vi "ExposeMapperToObjectNamepathDataRecursiverIterator.vi"(8 "BaseName":string, 9 "Skip Parent Name (t)":bool=TRUE, 11 "Value Reference In":refnum<data-value>) -> (2 "Object map":T1[](array[typedef]), 3 "Value Reference Out":refnum<data-value>)   [LabVIEW 2017]
uses:
  ExposeObjectMapNamepathData.ctl
  ExposeMapperDataTypeEnum.ctl
  ExposeObjectMapContainerTypeEnum.ctl
  ExposeMapperObjectTypeEnum.ctl
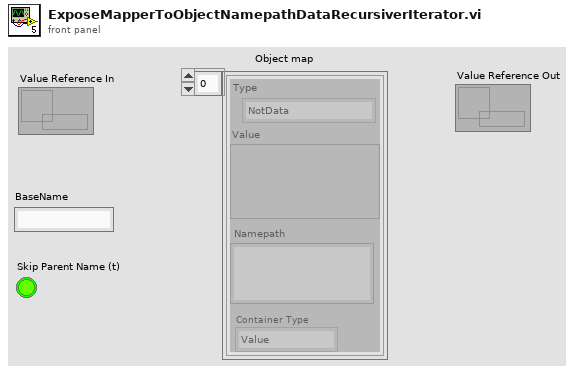
[diagram p1: front panel]
types:
  T1 = typedef "ExposeObjectMapNamepathData.ctl" = cluster{"Type":T2, "Value":variant, "Namepath":string, "Container Type":T3}
  T2 = typedef "ExposeMapperDataTypeEnum.ctl" = enum16{"NotData", "int8", "byte", "int16", "uint16", "int32", "uint32", "int64", "uint64", "Single", "Double", "String", "Boolean", "Container"}
  T3 = typedef "ExposeObjectMapContainerTypeEnum.ctl" = enum16{"Value", "Array", "Waveform", "NetContainer"}
  T4 = typedef "ExposeMapperObjectTypeEnum.ctl" = enum16{"NotAValidObject", "Value", "Variant", "Cluster", "Array", "Asng. Refnum"}
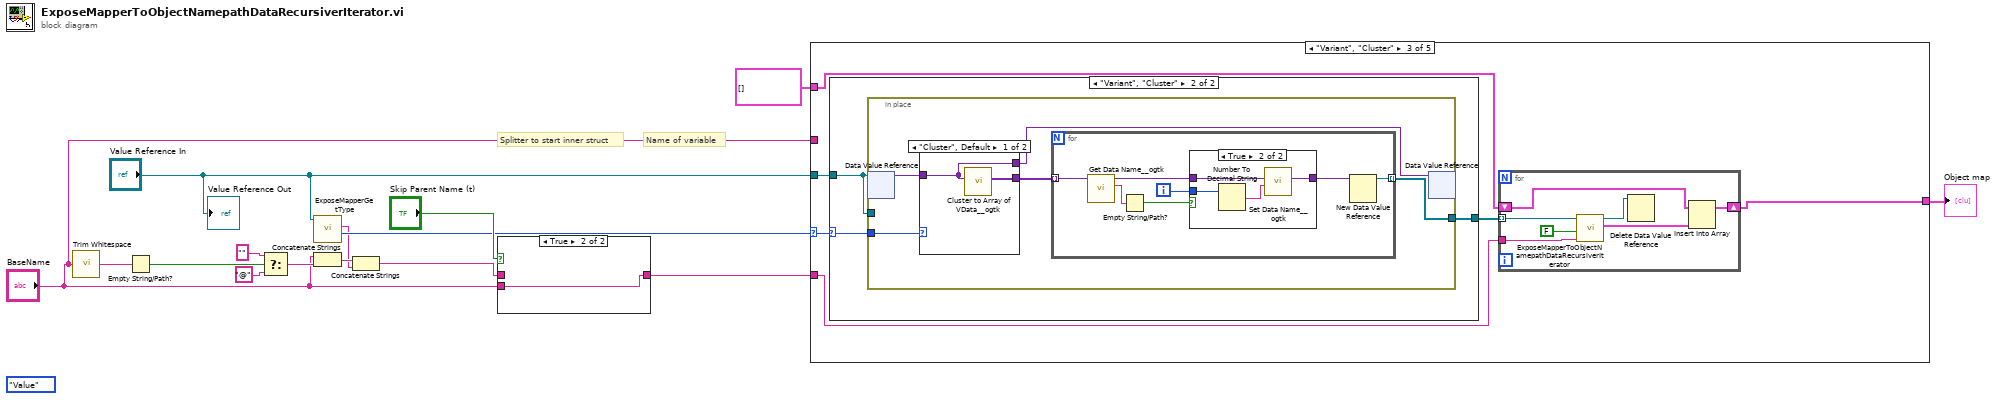
[diagram p0: block diagram]
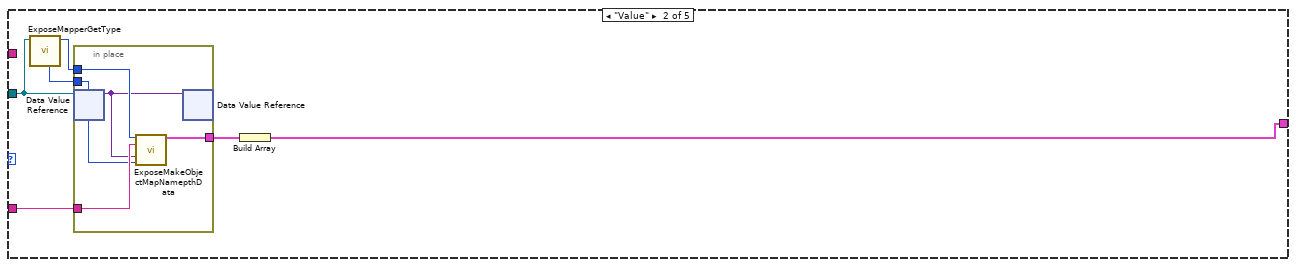
[diagram p4: hidden frame]
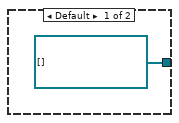
[diagram p5: hidden frame]
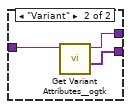
[diagram p6: hidden frame]
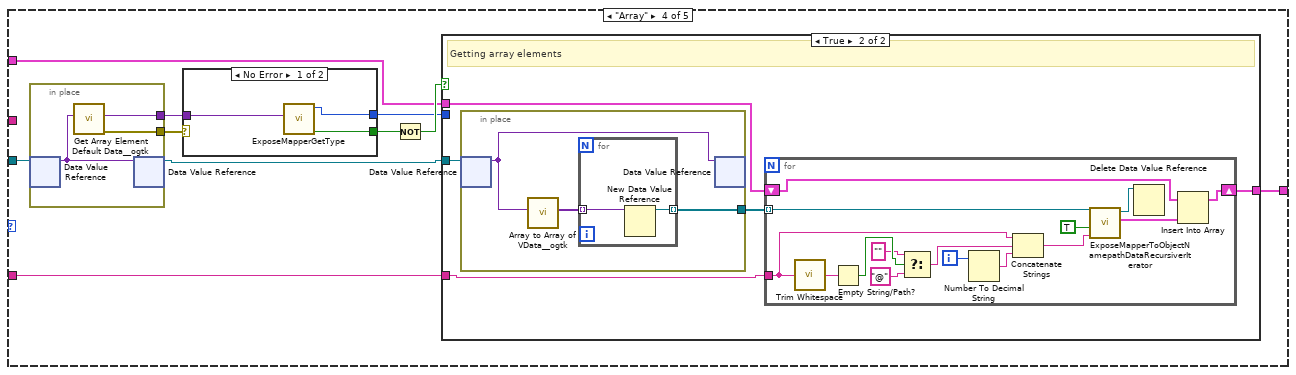
[diagram p8: hidden frame]
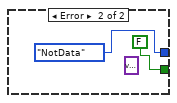
[diagram p9: hidden frame]
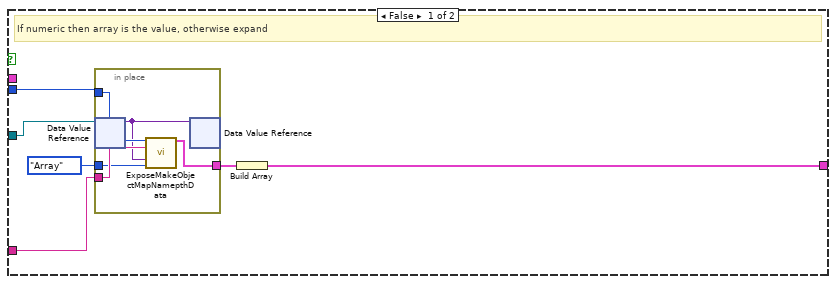
[diagram p10: hidden frame]
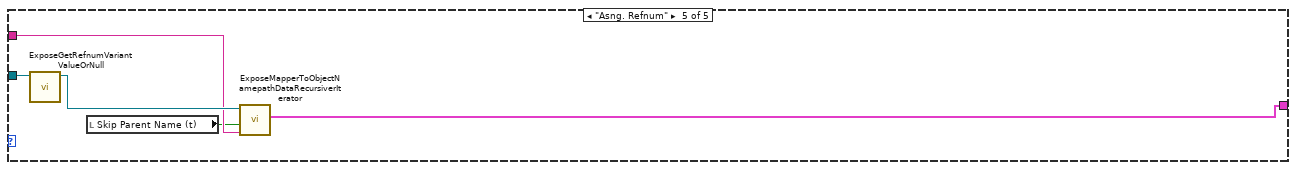
[diagram p11: hidden frame]
diagram:
  (unwired) ExposeMapperObjectTypeEnum."Value" ("OType")
  # "Splitter to start inner struct"
  # "Name of variable"
  n1 = call <vilib>:"Trim Whitespace.vi"("string"="BaseName") -> ("trimmed string"=w8:string)  [unwired: 1 in]
  n2 = Empty String/Path?(string/path=w8) -> (empty?=w7:bool)
  n3 = Select(t="" ("name"), s=w7, f="@" ("name")) -> (s? t:f=w15:string)
  n4 = call "ExposeMapperGetType.vi"("Data Val Ref in"="Value Reference In") -> ("OType"=w3:T4, "Name"=w2:string)  [unwired: 5 in, 4 out]
  n5 = Concatenate Strings("BaseName", w15) -> (w9:string)
  n6 = Concatenate Strings(w9, w2) -> (w11:string)
  n7 = case shown="True" "Skip Parent Name (t)" {
    tunnel: [w16 w17] -> w12
    tunnel: w11 -> [w16 _]
    tunnel: "BaseName" -> [_ w17]
    frame False {
    }
    frame True {
    }
  }
  n8 = case shown="\"Variant\", \"Cluster\"" w3 {
    selector: w3 -> [_ _ w31 _ _]
    tunnel: [w18 w23 w35 w78 w123] -> w5
    tunnel: w12 -> [_ w21 w34 w75 _]
    tunnel: "BaseName" -> [_ _ _ _ w126]
    tunnel: T1[] [] -> [w18 _ w33 w74 _]
    tunnel: "Value Reference In" -> [_ w19 w32 w70 w125]
    frame Default {
    }
    frame "Value" {
      n9 = call "ExposeMapperGetType.vi"("Data Val Ref in"=w19) -> ("DataType"=w22:T2, "Container Type (Labview Value type)"=w20:T3)  [unwired: 5 in, 4 out]
      n10 = in-place {
        in-place-border: [w29] -> w24
        in-place-border: w22 -> [w28]
        in-place-border: w21 -> [w27]
        in-place-border: w20 -> [w26]
        n11 = in-place-dvr #1(w19) -> (w25:variant)  [unwired: 1 out]
        n12 = call "ExposeMakeObjectMapNamepthData.vi"("ObjectMapType"=w28, "namepath"=w27, "value"=w25, "Labview Contriner type"=w26) -> ("MatlabDataBundle"=w29:T1)  [unwired: 11 in]
        n13 = in-place-dvr #1(w25) -> ()  [unwired: 2 out]
      }
      n14 = Build Array(w24) -> (w23:T1[])
    }
    frame "Variant", "Cluster" {
      n15 = case shown="\"Variant\", \"Cluster\"" w31 {
        selector: w31 -> [_ w37]
        tunnel: w32 -> [_ w39]
        tunnel: [refnum<data-value>[] [] w38] -> w30
        frame Default {
        }
        frame "Variant", "Cluster" {
          n16 = in-place {
            in-place-border: w39 -> [_]
            in-place-border: [w42] -> w38
            in-place-border: w37 -> [w40]
            n17 = in-place-dvr #2(w39) -> (w44:variant)  [unwired: 1 out]
            n18 = case shown="\"Cluster\", Default" w40 {
              tunnel: w44 -> [w46 w49]
              tunnel: [w45 w48] -> w43
              tunnel: [w46 w47] -> w41
              frame "Cluster", Default {
                n19 = call <userlib>:"Cluster to Array of VData__ogtk.vi"("Cluster"=w46) -> ("Array of VData"=w45:variant[])  [unwired: 9 in, 1 out]
              }
              frame "Variant" {
                n20 = call <userlib>:"Get Variant Attributes__ogtk.vi"("Variant"=w49) -> ("value(s)"=w48:variant[], "duplicate Variant"=w47:variant)  [unwired: 3 in, 2 out]
              }
            }
            n21 = for {
              tunnel: w43 -> [w55] mode=indexing
              tunnel: [w56] -> w42 mode=indexing
              i -> [w50]
              n22 = call <userlib>:"Get Data Name__ogtk.vi"("Data"=w55) -> ("Data Name"=w54:string, "Data dup"=w52:variant)  [unwired: 8 in, 1 out]
              n23 = Empty String/Path?(string/path=w54) -> (empty?=w53:bool)
              n24 = case shown="True" w53 {
                tunnel: w52 -> [w57 w60]
                tunnel: [w57 w59] -> w51
                tunnel: w50 -> [_ w61]
                frame False {
                }
                frame True {
                  n25 = Number To Decimal String(number=w61) -> (decimal integer string=w58:string)  [unwired: 1 in]
                  n26 = call <userlib>:"Set Data Name__ogtk.vi"("Data Name"=w58, "Data"=w60) -> ("Renamed Data"=w59:variant)  [unwired: 8 in, 1 out]
                }
              }
              n27 = New Data Value Reference(data value=w51) -> (data value reference=w56:refnum<data-value>)  [unwired: 1 in, 1 out]
            }
            n28 = in-place-dvr #2(w41) -> ()  [unwired: 2 out]
          }
        }
      }
      n29 = for {
        shift-right: [w68] -> w35
        shift-left: w33 -> [w66]
        tunnel: w34 -> [w67]
        tunnel: w30 -> [w63] mode=indexing
        n30 = call "ExposeMapperToObjectNamepathDataRecursiverIterator.vi"("BaseName"=w67, "Skip Parent Name (t)"=FALSE ("IgnoreContainerName"), "Value Reference In"=w63) -> ("Object map"=w64:T1[], "Value Reference Out"=w62:refnum<data-value>)  [unwired: 7 in]
        n31 = Delete Data Value Reference(data value reference=w62) -> ()  [unwired: 1 in, 2 out]
        n32 = Insert Into Array(array=w66, new element=w64) -> (w68:T1[])  [unwired: 1 in]
      }
    }
    frame "Array" {
      n33 = in-place {
        in-place-border: [w81] -> w73
        in-place-border: [w80] -> w71
        n34 = in-place-dvr #3(w70) -> (w79:variant)  [unwired: 1 out]
        n35 = call <userlib>:"Get Array Element Default Data__ogtk.vi"("Array"=w79) -> ("error out"=w81:errorcluster, "Array Element Default Data"=w80:variant)  [unwired: 9 in]
        n36 = in-place-dvr #3(w79) -> (w69:refnum<data-value>)  [unwired: 1 out]
      }
      n37 = case shown="No Error" w73 {
        tunnel: [w84 FALSE ("IsNumeric")] -> w77
        tunnel: [w83 ExposeMapperDataTypeEnum."NotData" ("MatlabType")] -> w72
        tunnel: w71 -> [w82 _]
        frame No Error {
          n38 = call "ExposeMapperGetType.vi"("Value"=w82) -> ("IsNumeric"=w84:bool, "DataType"=w83:T2)  [unwired: 5 in, 4 out]
        }
        frame Error {
          (unwired) variant
        }
      }
      n39 = Not(x=w77) -> (.not. x?=w76:bool)
      n40 = case shown="True" w76 {
        tunnel: [w90 w102] -> w78
        tunnel: w75 -> [w92 w101]
        tunnel: w74 -> [_ w100]
        tunnel: w69 -> [w87 w98]
        tunnel: w72 -> [w89 _]
        frame False {
          # "If numeric then array is the value, otherwise expand"
          n41 = in-place {
            in-place-border: w92 -> [w97]
            in-place-border: [w96] -> w91
            in-place-border: w89 -> [w95]
            in-place-border: ExposeObjectMapContainerTypeEnum."Array" ("Labview Contriner type") -> [w94]
            n42 = in-place-dvr #4(w87) -> (w93:variant)  [unwired: 1 out]
            n43 = call "ExposeMakeObjectMapNamepthData.vi"("ObjectMapType"=w95, "namepath"=w97, "value"=w93, "Labview Contriner type"=w94) -> ("MatlabDataBundle"=w96:T1)  [unwired: 11 in]
            n44 = in-place-dvr #4(w93) -> ()  [unwired: 2 out]
          }
          n45 = Build Array(w91) -> (w90:T1[])
        }
        frame True {
          # "Getting array elements"
          n46 = in-place {
            in-place-border: [w103] -> w99
            n47 = in-place-dvr #5(w98) -> (w105:variant)  [unwired: 1 out]
            n48 = call <userlib>:"Array to Array of VData__ogtk.vi"("MultiD Array"=w105) -> ("1D Array of Variants"=w104:variant[])  [unwired: 9 in, 1 out]
            n49 = for {
              tunnel: w104 -> [w107] mode=indexing
              tunnel: [w106] -> w103 mode=indexing
              n50 = New Data Value Reference(data value=w107) -> (data value reference=w106:refnum<data-value>)  [unwired: 1 in, 1 out]
            }
            n51 = in-place-dvr #5(w105) -> ()  [unwired: 2 out]
          }
          n52 = for {
            shift-right: [w122] -> w102
            shift-left: w100 -> [w118]
            tunnel: w101 -> [w115]
            tunnel: w99 -> [w110] mode=indexing
            i -> [w117]
            n53 = call <vilib>:"Trim Whitespace.vi"("string"=w115) -> ("trimmed string"=w116:string)  [unwired: 1 in]
            n54 = Empty String/Path?(string/path=w116) -> (empty?=w114:bool)
            n55 = Select(t="", s=w114, f="@" ("string")) -> (s? t:f=w111:string)
            n56 = Number To Decimal String(number=w117) -> (decimal integer string=w121:string)  [unwired: 1 in]
            n57 = Concatenate Strings(w115, w111, w121) -> (w120:string)
            n58 = call "ExposeMapperToObjectNamepathDataRecursiverIterator.vi"("BaseName"=w120, "Skip Parent Name (t)"=TRUE ("IgnoreContainerName"), "Value Reference In"=w110) -> ("Object map"=w108:T1[], "Value Reference Out"=w109:refnum<data-value>)  [unwired: 7 in]
            n59 = Delete Data Value Reference(data value reference=w109) -> ()  [unwired: 1 in, 2 out]
            n60 = Insert Into Array(array=w118, new element=w108) -> (w122:T1[])  [unwired: 1 in]
          }
        }
      }
    }
    frame "Asng. Refnum" {
      n61 = call "ExposeGetRefnumVariantValueOrNull.vi"("Data Value Reference in"=w125) -> ("Data Value Reference Out"=w127:refnum<data-value>)  [unwired: 8 in, 2 out]
      n62 = local read "Skip Parent Name (t)"() -> (w124:bool)
      n63 = call "ExposeMapperToObjectNamepathDataRecursiverIterator.vi"("BaseName"=w126, "Skip Parent Name (t)"=w124, "Value Reference In"=w127) -> ("Object map"=w123:T1[])  [unwired: 7 in, 1 out]
    }
  }
  "Object map" <- w5
  "Value Reference Out" <- "Value Reference In"
